vi "gfitsio-read-key-datetime.vi"(7 "keyname":string, 8 "error in (no error)":errorcluster, 9 "default value":timestamp, 11 "gfits refnum":T1) -> (0 "error out":errorcluster, 1 "comment":string, 2 "value":timestamp, 3 "dup gfits refnum":T1)   [LabVIEW 2019, in "gfitsio.lvlib"]
doc: "Return the specified keyword. <B>default value</B> specifies the desired returned data type of the keyword value. Data type conversion will be performed for numeric values if the keyword value does not have the same data type. If the keyword does not exist or an error occurs <B>value</B> will be equal to <B>default value</B>."
uses:
  gfitsio.lvlib
  gfitsio-refnum.ctl
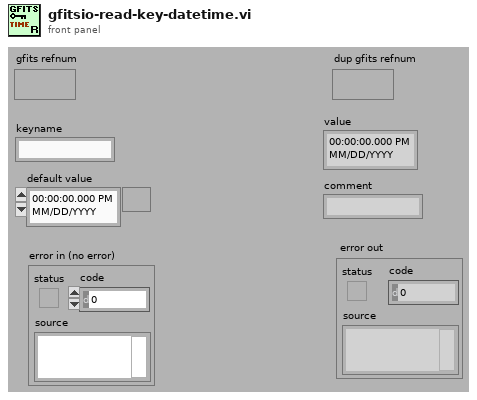
[diagram p1: front panel]
types:
  T1 = typedef "gfitsio.lvlib/gfitsio-refnum.ctl" = refnum<k1>
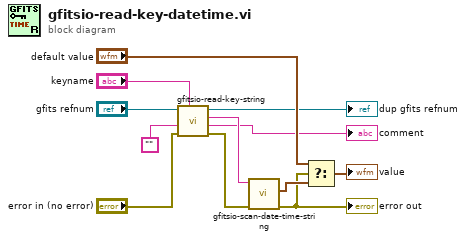
[diagram p0: block diagram]
diagram:
  n1 = call "gfitsio-read-key-string.vi"("keyname"="keyname", "error in (no error)"="error in (no error)", "default value"="", "gfits refnum"="gfits refnum") -> ("error out"=w4:errorcluster, "comment"=→"comment":string, "value"=w3:string, "dup gfits refnum"=→"dup gfits refnum":T1)  [unwired: 1 in, 3 out]
  n2 = call "gfitsio-scan-date-time-string.vi"("error in (no error)"=w4, "date/time string"=w3) -> ("error out"=w11:errorcluster, "timestamp"=w12:timestamp)  [unwired: 8 out]
  "error out" <- w11
  n3 = Select(t="default value", s=w11, f=w12) -> (s? t:f=→"value":timestamp)
